vi "_Request StringList with lvcsm Support.vi"(5 "API Ref":refnum<vi>, 6 "Config Path (\"\" For Lvcsm File)":path, 7 "Current Module (\"\" to Generate an ID)":string, 8 "error in (no error)":errorcluster, 9 "Force? (F)":bool, 10 "API Name":string="CSMAPI", 11 "CSM Name":string) -> (0 "error out":errorcluster, 3 "CSMAPI List":string[](array[string]))   [LabVIEW 2017, in "CSM-Helper API with lvcsm Support.lvlib"]
uses:
  CSM-Helper.lvclass
  b7efc127-9b6c-49b9-9e9d-39643bcb625b.vi
  166189b3-b0ee-4f88-bea7-bb947d9812ee.vi
  913c550f-f939-4955-8b9d-1380e6caaad2.vi
  b420853c-3190-4e75-95ae-0734db192402.vi
  <vilib>/Utility/config.llb/Close Config Data.vi
  <vilib>/Utility/config.llb/Write Key.vi
  <vilib>/Utility/config.llb/Write Key (Double).vi
  <vilib>/Utility/config.llb/Write Key (I32).vi
  <vilib>/Utility/config.llb/Write Key (String).vi
  lvcsmFile/Path to lvcsm String.vi
  <vilib>/Utility/config.llb/Remove Key.vi
  <vilib>/Utility/config.llb/Get Key Names.vi
  <vilib>/Utility/Data Type/Get Type Information.vi
  <vilib>/Utility/Data Type/Get Array Information.vi
  <vilib>/Utility/config.llb/Write Key (Boolean).vi
  <vilib>/Utility/config.llb/Open Config Data.vi
  lvcsmFile/lvcsm File Path.vi
  lvcsmFile/_Array of VData to VCluster.vi
  <vilib>/Utility/config.llb/Read Key.vi
  <vilib>/Utility/config.llb/Read Key (Double).vi
  <vilib>/Utility/config.llb/Read Key (I32).vi
  lvcsmFile/lvcsm String to Path.vi
  <vilib>/Utility/config.llb/Read Key (String).vi
  <vilib>/Utility/config.llb/Read Key (Boolean).vi
  API/Create From VI Reference.vi
  API/Destroy.vi
  CSM-Helper API with lvcsm Support.lvlib
  Communicable State Machine.lvlib
  Properties/Read APIs.vi
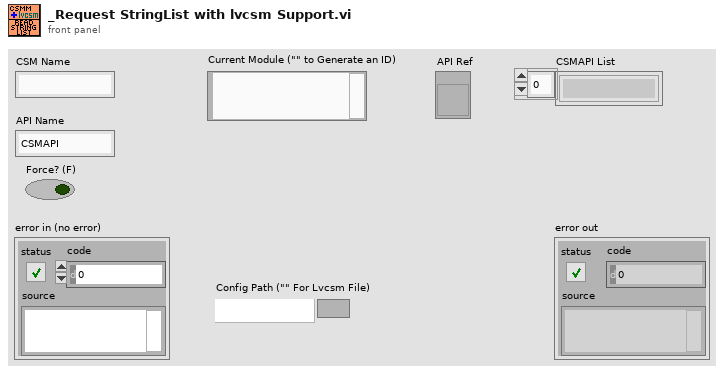
[diagram p1: front panel]
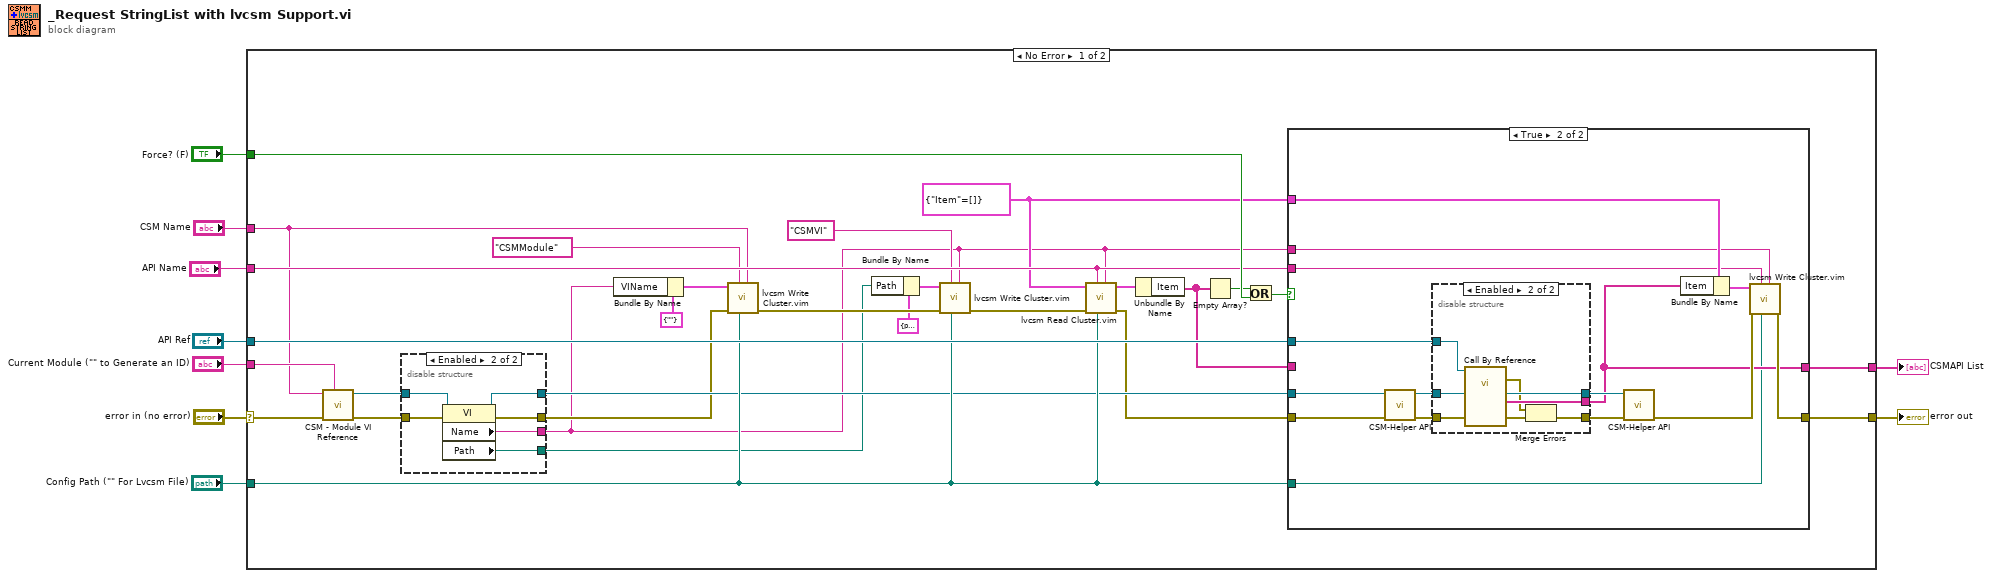
[diagram p0: block diagram]
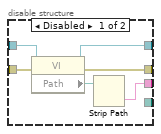
[diagram p2: hidden frame]
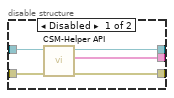
[diagram p4: hidden frame]
diagram:
  n1 = case shown="No Error" "error in (no error)" {
    selector: "error in (no error)" -> [w37 w81]
    tunnel: [w38 w81] -> w9
    tunnel: "CSM Name" -> [w31 _]
    tunnel: "Current Module (\"\" to Generate an ID)" -> [w36 _]
    tunnel: [w35 _] -> w5
    tunnel: "Force? (F)" -> [w34 _]
    tunnel: "Config Path (\"\" For Lvcsm File)" -> [w30 _]
    tunnel: "API Ref" -> [w33 _]
    tunnel: "API Name" -> [w32 _]
    frame No Error {
      w23 = cluster{"Item":string[]} {"Item"=[]}
      n2 = call "CSM - Module VI Reference.vi"("Current Module (\"\" to Generate an ID)"=w36, "error in (no error)"=w37, "CSM Name"=w31) -> ("error out"=w29:errorcluster, "CSM Module VIRef"=w28:refnum<vi>)  [unwired: 7 in]
      n3 = disable-structure shown="Enabled" {
        disable-tunnel: w29 -> [w44 w50]
        disable-tunnel: w28 -> [w43 w49]
        disable-tunnel: [w42 w48] -> w27
        disable-tunnel: [w40 w47] -> w20
        disable-tunnel: [w39 w46] -> w13
        disable-tunnel: [_ w45] -> w10
        frame Disabled {
          n4 = property class="VI"(reference=w43, error in=w44) -> (reference out=w42:refnum<vi>, error out=w40:errorcluster, "Path"=w41:path)
          n5 = Strip Path(path=w41) -> (name=w39:string)  [unwired: 1 out]
        }
        frame Enabled {
          n6 = property class="VI"(reference=w49, error in=w50) -> (reference out=w48:refnum<vi>, error out=w47:errorcluster, "Name"=w46:string, "Path"=w45:path)
        }
      }
      n7 = Bundle By Name(cluster=cluster{"VIName":string} {"VIName"=""}, "VIName"=w13) -> (w17:cluster{"VIName":string})
      n8 = call "lvcsm Write Cluster.vim"("Sub-section (\"\")"=w31, "Config Path"=w30, "Section"="CSMModule", "Error In"=w20, "Configuration"=w17) -> ("error out"=w16:errorcluster)  [unwired: 6 in]
      n9 = Bundle By Name(cluster=cluster{"Path":path} {"Path"=path ""}, "Path"=w10) -> (w12:cluster{"Path":path})
      n10 = call "lvcsm Write Cluster.vim"("Sub-section (\"\")"=w13, "Config Path"=w30, "Section"="CSMVI", "Error In"=w16, "Configuration"=w12) -> ("error out"=w15:errorcluster)  [unwired: 6 in]
      n11 = call "lvcsm Read Cluster.vim"("Sub-section (\"\")"=w13, "Config Path"=w30, "Section"=w32, "Error In"=w15, "Default Prototype"=w23) -> ("error out"=w24:errorcluster, "Cluster (Dup)"=w26:cluster{"Item":string[]})  [unwired: 5 in]
      n12 = Unbundle By Name(w26) -> ("Item"=w22:string[])
      n13 = Empty Array?(array=w22) -> (empty?=w25:bool)
      n14 = Or(x=w25, y=w34) -> (x .or. y?=w21:bool)
      n15 = case shown="True" w21 {
        tunnel: w24 -> [w52 w63]
        tunnel: w27 -> [_ w62]
        tunnel: [w52 w58] -> w38
        tunnel: w23 -> [_ w61]
        tunnel: w32 -> [_ w57]
        tunnel: w13 -> [_ w56]
        tunnel: [w51 w55] -> w35
        tunnel: w22 -> [w51 _]
        tunnel: w30 -> [_ w54]
        tunnel: w33 -> [_ w53]
        frame False {
        }
        frame True {
          n16 = call-poly "CSM-Helper API.vi"("error in (no error)"=w63, "VI"=w62) -> ("error out"=w65:errorcluster, "CSM-Helper.lvclass"=w64:refnum<class "CSM-Helper.lvclass">)  [unwired: 8 in]
          n17 = disable-structure shown="Enabled" {
            disable-tunnel: [w72 w74] -> w67
            disable-tunnel: [w71 w78] -> w66
            disable-tunnel: w65 -> [w70 w77]
            disable-tunnel: w64 -> [w69 w79]
            disable-tunnel: [w68 w75] -> w55
            disable-tunnel: w53 -> [_ w80]
            frame Disabled {
              n18 = call-poly "CSM-Helper API.vi"("error in (no error)"=w70, "CSM-Helper in"=w69) -> ("error out"=w72:errorcluster, "Value"=w68:string[], "CSM-Helper out"=w71:refnum<class "CSM-Helper.lvclass">)  [unwired: 7 in]
            }
            frame Enabled {
              n19 = call-by-ref "?"(reference=w80, "error in (no error)"=w77, "CSM-Helper in"=w79) -> (error out=w73:errorcluster, 0:"error out"=w76:errorcluster, "Value"=w75:string[], "CSM-Helper out"=w78:refnum<class "CSM-Helper.lvclass">)  [unwired: 8 in, 1 out]
              n20 = Merge Errors(w73, w76) -> (w74:errorcluster)
            }
          }
          n21 = call-poly "CSM-Helper API.vi"("error in (no error)"=w67, "CSM-Helper in"=w66) -> ("error out"=w59:errorcluster)  [unwired: 8 in, 1 out]
          n22 = Bundle By Name(cluster=w61, "Item"=w55) -> (w60:cluster{"Item":string[]})
          n23 = call "lvcsm Write Cluster.vim"("Sub-section (\"\")"=w56, "Config Path"=w54, "Section"=w57, "Error In"=w59, "Configuration"=w60) -> ("error out"=w58:errorcluster)  [unwired: 6 in]
        }
      }
    }
    frame Error {
    }
  }
  "error out" <- w9
  "CSMAPI List" <- w5
